vi "ROI entry-Load dataset.vi"(8 "error in (no error)":errorcluster, 11 "Experiment folder path OR Z-stack folder path":path) -> (0 "error out":errorcluster)   [LabVIEW 2017]
uses:
  Typedefs/ROI management FG states.ctl
  Global Variables/General Globals.vi
  ROI Entry screen/Globals/gl_ROI Entry UI globals.vi
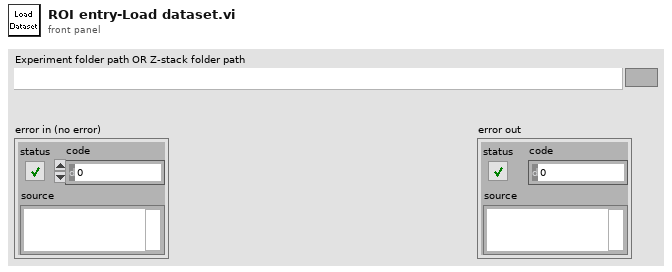
[diagram p1: front panel]
types:
  T1 = typedef "ROI management FG states.ctl" = enum16{"Read", "Write", "Write-from dataset", "Clear Last", "Clear All", "Update ROIs time", "Reload last ROI set", "Offset all ROI", "Offset visible ROI"}
  T2 = typedef "IMAQ Image.ctl" = refnum<image>
  T3 = cluster{"RedImageArray":T2[], "GreenImageArray":T2[], "RedMaxZ":T2, "GreenMaxZ":T2, "AOL Z Planes":dbl[], "AOL Z Planes (norm)":dbl[], "Motor Z planes":dbl[]}
  T4 = typedef "ROI entry screen ctrl refs cluster.ctl" = cluster{"Done button":refnum<vi>, "Imaging button":refnum<vi>, "Acquisition button":refnum<vi>, "POI dwell time (us)":refnum<vi>, "Scan dwell time per pixel (us)":refnum<vi>, "# of planes":refnum<vi>, "Zoom Ctrl":refnum<vi>, "Equal size":refnum<vi>, "Channel":refnum<vi>, "Image Display":refnum<vi>, "Z-Plane Selector":refnum<vi>, "Number of lines left":refnum<vi>, "Z-stack folder path":refnum<vi>, "POI Density":refnum<vi>, "Arb Plane Entry":refnum<vi>, "Whole plane":refnum<vi>, "Clear Last":refnum<vi>, "Clear All":refnum<vi>, "Trial Length (sec)":refnum<vi>, "Palette Type":refnum<vi>, "Intensity slider":refnum<vi>, "# POI":refnum<vi>, "Max Z Proj":refnum<vi>, "Zplane ind":refnum<vi>, "Wavelength (nm)":refnum<vi>, "Number of Trials":refnum<vi>, "Funct stim.trig.enable":refnum<vi>, "Funct stim.trig.delay (s)":refnum<vi>, "Line Mode":refnum<vi>, "Step size (µm)":refnum<vi>, "ROI move mode":refnum<vi>, "Cool-down time (s)":refnum<vi>, "Enable cool-down time":refnum<vi>, "Motor Z ind. (um)":refnum<vi>, "AOL Z ind. (um)":refnum<vi>, "Load Reference Image":refnum<vi>}
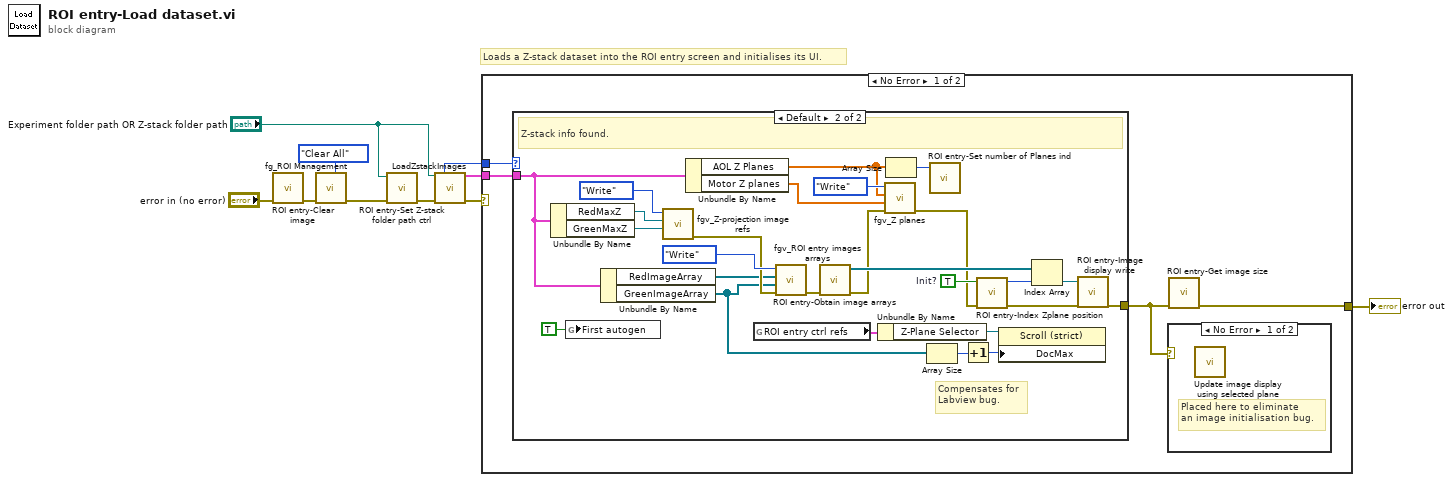
[diagram p0: block diagram]
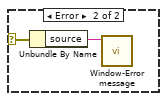
[diagram p2: hidden frame]
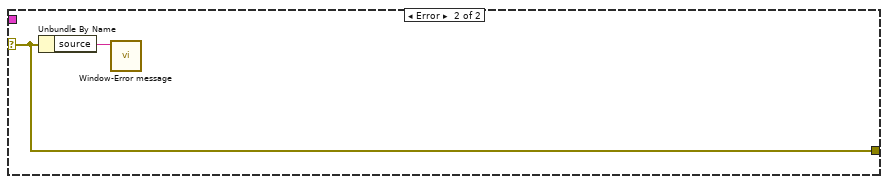
[diagram p4: hidden frame]
diagram:
  # "Loads a Z-stack dataset into the ROI entry screen and initialises its UI."
  n1 = call "ROI entry-Clear image.vi"("error in (no error)"="error in (no error)") -> ("error out"=w9:errorcluster)  [unwired: 10 in]
  n2 = call "fg_ROI Management.vi"("Function"=ROI_management_FG_states."Clear All", "error in (no error)"=w9) -> ("error out"=w3:errorcluster)  [unwired: 4 in, 5 out]
  n3 = call "ROI entry-Set Z-stack folder path ctrl.vi"("error in (no error)"=w3, "Experiment folder path OR Z-stack images folder path"="Experiment folder path OR Z-stack folder path") -> ("error out"=w1:errorcluster)  [unwired: 9 in]
  n4 = call "LoadZstackImages.vi"("Experiment folder path OR Z-stack folder path"="Experiment folder path OR Z-stack folder path", "error in (no error)"=w1) -> ("Number of Files"=w5:i32, "All outputs"=w7:T3, "Error Out"=w6:errorcluster)  [unwired: 4 in, 7 out]
  n5 = case shown="No Error" w6 {
    selector: w6 -> [_ w42]
    tunnel: w5 -> [w14 _]
    tunnel: w7 -> [w13 _]
    tunnel: [w12 w42] -> w4
    frame No Error {
      n6 = case shown="Default" w14 {
        tunnel: w13 -> [_ w21]
        tunnel: [_ w17] -> w11
        frame ..0 {
          # "Number of planes <=0 (i.e. Z-stack info not found.)"
        }
        frame Default {
          w33 = TRUE  # Init?
          # "Compensates for Labview bug."
          # "Z-stack info found."
          n7 = Unbundle By Name(w21) -> ("RedMaxZ"=w20:T2, "GreenMaxZ"=w19:T2)
          n8 = global write "General Globals.vi" "First autogen"(TRUE ("First autogen")) -> ()
          n9 = Unbundle By Name(w21) -> ("RedImageArray"=w22:T2[], "GreenImageArray"=w18:T2[])
          n10 = call "fgv_Z-projection image refs.vi"("GreenMaxZ"=w19, "RedMaxZ"=w20, "Function"=enum16{"Intialize", "Write", "Read", "Clear"}."Write") -> ("error out"=w27:errorcluster)  [unwired: 6 in, 2 out]
          n11 = Unbundle By Name(w21) -> ("AOL Z Planes"=w24:dbl[], "Motor Z planes"=w23:dbl[])
          n12 = global read "gl_ROI Entry UI globals.vi" "ROI entry ctrl refs"() -> (w30:T4)
          n13 = call "fgv_ROI entry images arrays.vi"("error in (no error)"=w27, "GreenImageArray"=w18, "RedImageArray"=w22, "Function"=enum16{"Intialize", "Write", "Read", "Clear"}."Write") -> ("error out"=w36:errorcluster)  [unwired: 5 in, 2 out]
          n14 = call "ROI entry-Obtain image arrays.vi"("error in (no error)"=w36) -> ("error IO"=w26:errorcluster, "RedImageArray"=w41:T2[])  [unwired: 9 in]
          n15 = Unbundle By Name(w30) -> ("Z-Plane Selector"=w31:refnum<vi>)
          n16 = call "fgv_Z planes.vi"("error in (no error)"=w26, "Motor Z planes"=w23, "AOL Z Planes"=w24, "Function"=enum16{"Intialize", "Write", "Read", "Clear"}."Write") -> ("error out"=w25:errorcluster)  [unwired: 5 in, 2 out]
          n17 = Array Size(array=w24) -> (size(s)=w32:i32)
          n18 = Array Size(array=w18) -> (size(s)=w39:i32)
          n19 = call "ROI entry-Set number of Planes ind.vi"("# of Z-Planes"=w32) -> ()  [unwired: 10 in, 1 out]
          n20 = Increment(x=w39) -> (x+1=w29:i32)
          n21 = call "ROI entry-Index Zplane position.vi"("error in (no error)"=w25, "Init?"=w33) -> ("error out"=w17:errorcluster, "Z-plane selector (index)"=w40:i32)  [unwired: 8 in]
          n22 = property on="Property Node" class="Scroll (strict)"(reference=w31, "DocMax"=w29) -> ()  [unwired: 1 in, 2 out]
          n23 = Index Array(array=w41, index=w40) -> (element=w38:T2)
          n24 = call "ROI entry-Image display write.vi"("Value"=w38) -> ()  [unwired: 4 in, 1 out]
        }
      }
      n25 = case shown="No Error" w11 {
        selector: w11 -> [_ w15]
        frame No Error {
          # "Placed here to eliminate\nan image initialisation bug."
          n26 = call "Update image display using selected plane.vi"() -> ()  [unwired: 11 in, 1 out]
        }
        frame Error {
          n27 = Unbundle By Name(w15) -> ("source"=w16:string)
          n28 = call "Window-Error message.vi"("Message"=w16) -> ()  [unwired: 10 in, 1 out]
        }
      }
      n29 = call "ROI entry-Get image size.vi"("error in (no error)"=w11) -> ("error out"=w12:errorcluster)  [unwired: 9 in, 1 out]
    }
    frame Error {
      n30 = Unbundle By Name(w42) -> ("source"=w43:string)
      n31 = call "Window-Error message.vi"("Message"=w43) -> ()  [unwired: 10 in, 1 out]
    }
  }
  "error out" <- w4
